vi "Thread_Conductor.vi"(5 "Ce VI":refnum<vi>, 7 "Display":refnum<vi>, 8 "entrée d'erreur (pas d'erreur)":errorcluster, 11 "File d'attente en entrée":refnum<queue>) -> (0 "error out":errorcluster caption="sortie d'erreur", 2 "Data Cluster":T1, 3 "File d'attente en sortie":refnum<queue>)   [LabVIEW 2020]
doc: "Conductor thread qui va gérer les opération"
uses:
  support/Message Queue/Message Cluster.ctl
  controls/UI Data.ctl
  support/Message Queue/All Message Queues.ctl
  Calculatrice/controls/ctrl_UI_Ref.ctl
  Calculatrice/controls/ctrl_Ref.ctl
  Calculatrice/controls/ctrl_Event_Ref.ctl
  controls/Ctrl_RefPad.ctl
  support/Message Queue/Enqueue Message (Single).vi
  <vilib>/Utility/error.llb/Error Cluster From Error Code.vi
  <vilib>/ErrorRing/Error Ring.xnode
  support/Message Queue/Message Queue.lvlib
  support/User Event - Stop/User Event - Stop.lvlib
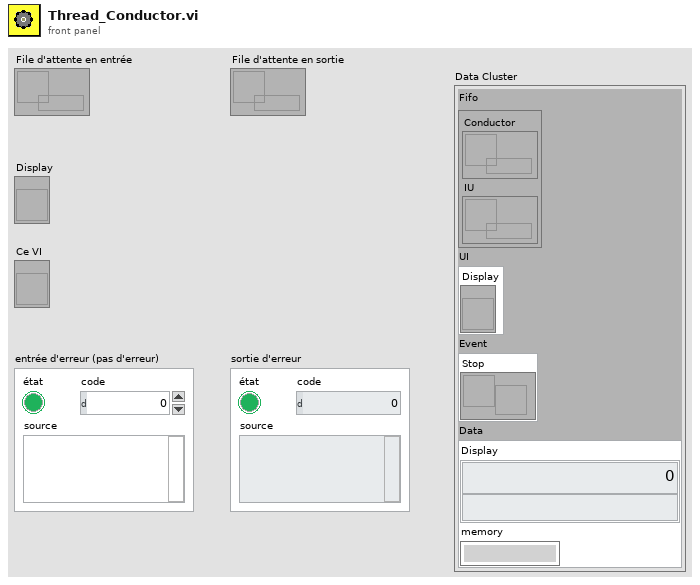
[diagram p1: front panel]
types:
  T1 = typedef "UI Data.ctl" = cluster{"Fifo":T2, "UI":T3, "Event":cluster{"Stop":refnum<user-event>}, "Data":cluster{"Display":cluster{"Num":dbl, "Char":string}, "memory":string}}
  T2 = typedef "Message Queue.lvlib/All Message Queues.ctl" = cluster{"Conductor":refnum<queue>, "IU":refnum<queue>}
  T3 = typedef "ctrl_UI_Ref.ctl" = cluster{"Display":refnum<vi>}
  T4 = typedef "ctrl_Ref.ctl" = cluster{"Fifo":T2, "Event":T5, "UI":T3}
  T5 = typedef "ctrl_Event_Ref.ctl" = cluster{"Stop Event":refnum<user-event>}
  T6 = typedef "Ctrl_RefPad.ctl" = cluster{"BTN_Ref":refnum<vi>, "CharPad":string}
  T7 = cluster{"état":bool, "code":i32, "source":string}
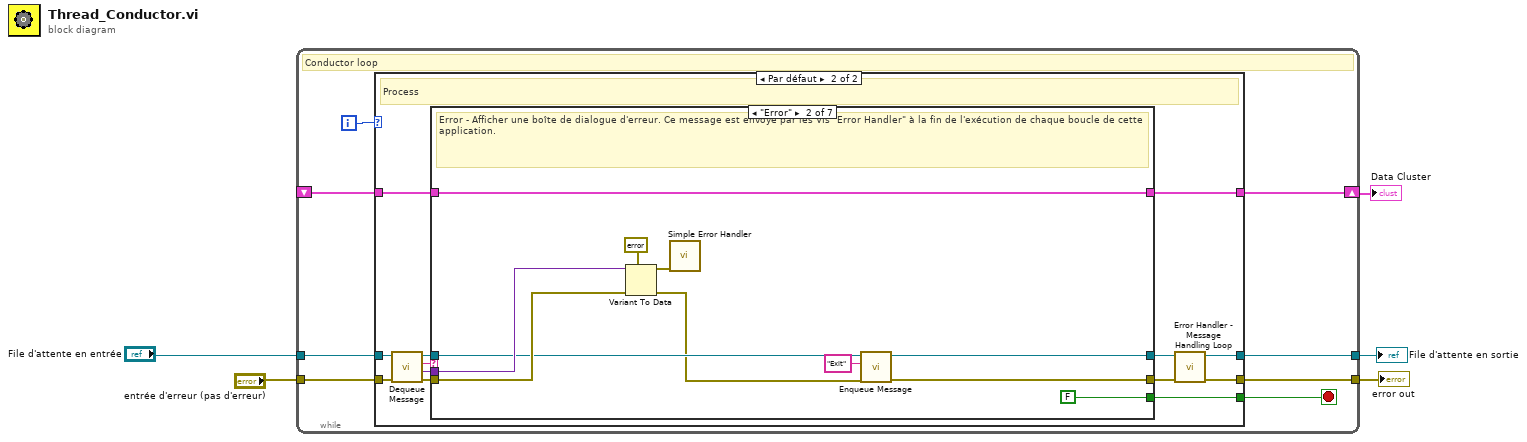
[diagram p0: block diagram]
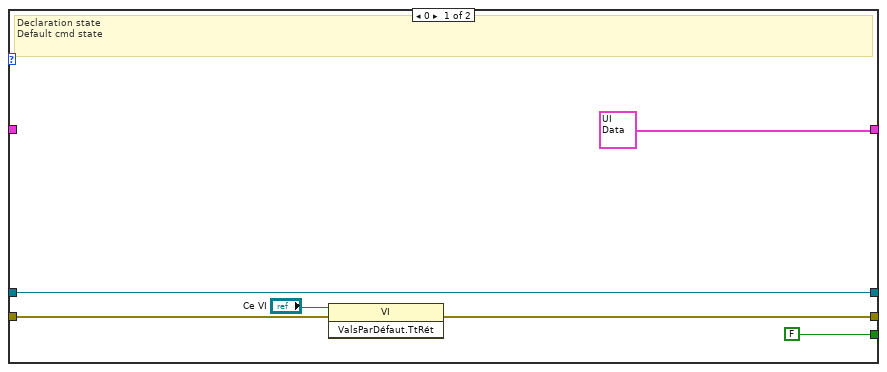
[diagram p2: hidden frame]
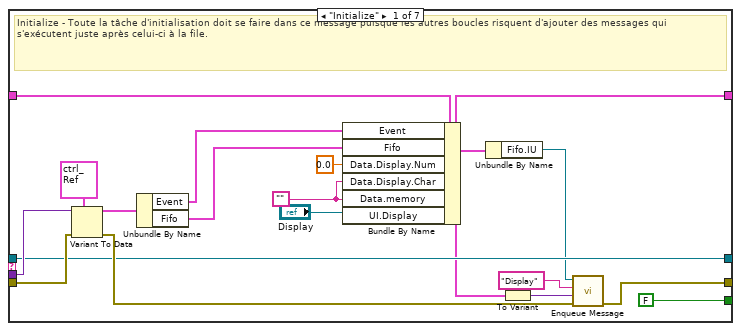
[diagram p3: hidden frame]
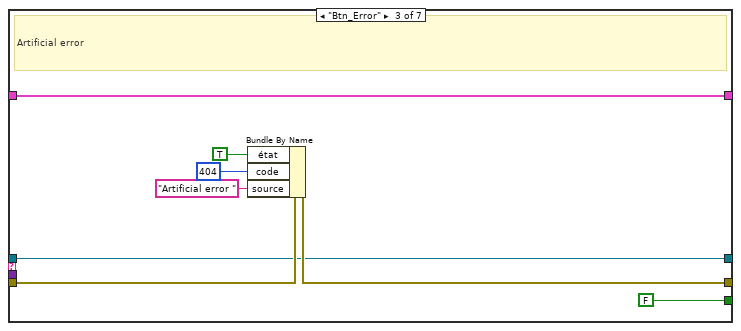
[diagram p4: hidden frame]
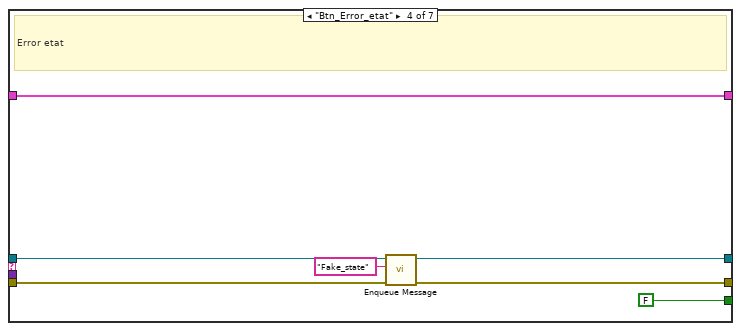
[diagram p5: hidden frame]
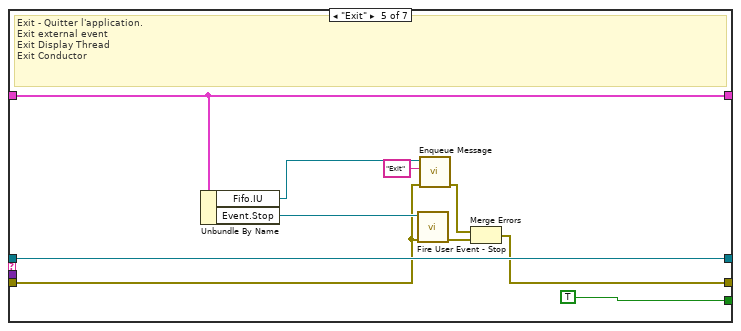
[diagram p6: hidden frame]
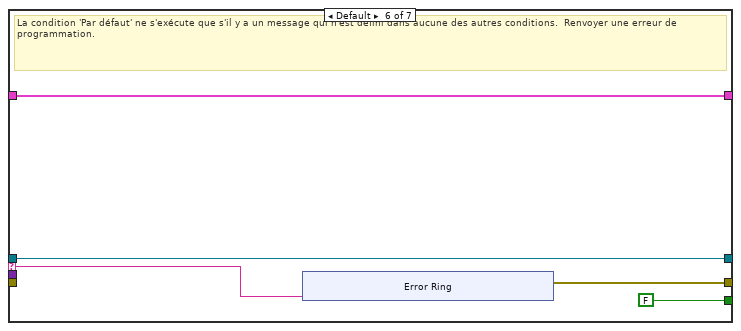
[diagram p7: hidden frame]
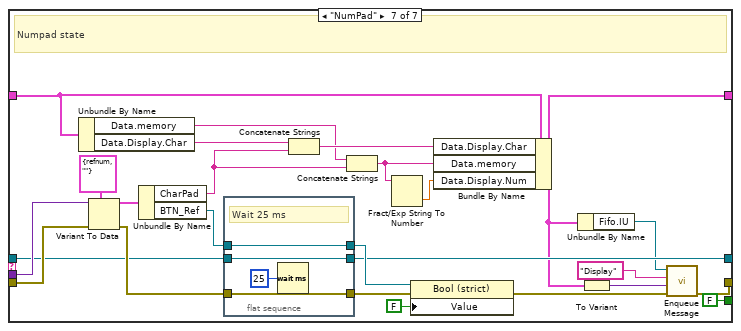
[diagram p8: hidden frame]
diagram:
  n1 = while {
    tunnel: "File d'attente en entrée" -> [w9]
    shift-right: [w12] -> w3
    shift-left: _ -> [w13]
    tunnel: "entrée d'erreur (pas d'erreur)" -> [w10]
    tunnel: [w8] -> w1
    tunnel: [w7] -> w4
    i -> [w6]
    stop <- w11 stop-if-true
    # "Conductor loop"
    n2 = case shown="Par défaut" w6 {
      tunnel: w13 -> [_ w32]
      tunnel: [T1 {"Fifo"={"Conductor"=refnum, "IU"=refnum}, "UI"={"Display"=refnum}, "Event"={"Stop"=refnum}, "Data"={"Display"={"Num"=0.0, "Char"=""}, "memory"=""}} ("Data Cluster") w31] -> w12
      tunnel: [FALSE w30] -> w11
      tunnel: w10 -> [w15 w29]
      tunnel: w9 -> [w18 w25]
      tunnel: [w14 w23] -> w8
      tunnel: [w18 w20] -> w7
      frame 0 {
        # "Declaration state\nDefault cmd state"
        n3 = invoke class="VI" method="ValsParDéfaut.TtRét"(reference="Ce VI", error in=w15) -> (error out=w14:errorcluster)  [unwired: 1 in, 2 out]
      }
      frame Default {
        # "Process"
        n4 = call "Dequeue Message.vi"("error in (no error)"=w29, "File d'attente de messages"=w25) -> ("error out"=w28:T7, "Données de message"=w26:variant, "Message"=w27:string, "File d'attente de message dup."=w24:refnum<queue>)  [unwired: 6 in]
        n5 = case "Conditions des messages" shown="\"Error\"" w27 {
          selector: w27 -> [_ _ _ _ _ w89 _]
          tunnel: w24 -> [w36 w55 w63 w72 w83 w87 w107]
          tunnel: w28 -> [w47 w61 w69 w75 w80 _ w123]
          tunnel: [w50 w52 w67 w74 w79 w90 w119] -> w22
          tunnel: w32 -> [w49 w60 w68 w76 w85 w91 w118]
          tunnel: [w34 w60 w68 w76 w85 w91 w100] -> w31
          tunnel: [FALSE FALSE FALSE FALSE TRUE FALSE FALSE] -> w30
          tunnel: w26 -> [w46 w59 _ _ _ _ w122]
          tunnel: [w36 w54 w63 w73 w83 w87 w101] -> w21
          frame "Initialize" {
            w43 = ""
            # "Initialize - Toute la tâche d'initialisation doit se faire dans ce message puisque les autres boucles risquent d'ajouter des messages qui s'exécutent juste après celui-ci à la file."
            n6 = Variant To Data(error in=w47, type=T4 {"Fifo"={"Conductor"=refnum, "IU"=refnum}, "Event"={"Stop Event"=refnum}, "UI"={"Display"=refnum}} ("Ref"), Variant=w46) -> (data=w40:T4, error out=w45:errorcluster)
            n7 = Unbundle By Name(w40) -> ("Event"=w38:T5, "Fifo"=w39:T2)
            n8 = Bundle By Name(cluster=w49, "Event"=w38, "Fifo"=w39, "Data.Display.Num"=0.0, "Data.Display.Char"=w43, "Data.memory"=w43, "UI.Display"="Display") -> (w34:T1)
            n9 = Unbundle By Name(w34) -> ("Fifo.IU"=w33:refnum<queue>)
            n10 = To Variant(anything=w34) -> (Variant=w35:variant)
            n11 = call-poly "Enqueue Message.vi"("error in (no error)"=w45, "Données de message"=w35, "Message"="Display", "File d'attente de messages"=w33) -> ("error out"=w50:T7)  [unwired: 6 in, 1 out]
          }
          frame "Error" {
            # "Error - Afficher une boîte de dialogue d'erreur. Ce message est envoyé par les VIs \"Error Handler\" à la fin de l'exécution de chaque boucle de cette application."
            n12 = Variant To Data(error in=w61, type=errorcluster {"status"=FALSE, "code"=0, "source"=""} ("error constant"), Variant=w59) -> (data=w57:errorcluster, error out=w53:errorcluster)
            n13 = call <vilib>:"Simple Error Handler.vi"("error in (no error)"=w57) -> ()  [unwired: 4 in, 5 out]
            n14 = call-poly "Enqueue Message.vi"("error in (no error)"=w53, "Message"="Exit", "File d'attente de messages"=w55) -> ("error out"=w52:T7, "File d'attente de message dup."=w54:refnum<queue>)  [unwired: 7 in]
          }
          frame "Btn_Error" {
            # "Artificial error"
            n15 = Bundle By Name(cluster=w69, "état"=TRUE, "code"=404, "source"="Artificial error ") -> (w67:T7)
          }
          frame "Btn_Error_etat" {
            # "Error etat"
            n16 = call-poly "Enqueue Message.vi"("error in (no error)"=w75, "Message"="Fake_state", "File d'attente de messages"=w72) -> ("error out"=w74:T7, "File d'attente de message dup."=w73:refnum<queue>)  [unwired: 7 in]
          }
          frame "Exit" {
            # "Exit - Quitter l'application.\nExit external event\nExit Display Thread\nExit Conductor"
            n17 = Unbundle By Name(w85) -> ("Fifo.IU"=w81:refnum<queue>, "Event.Stop"=w84:refnum<user-event>)
            n18 = call "Fire User Event - Stop.vi"("error in (no error)"=w80, "Événement utilisateur - Arrêt"=w84) -> ("error out"=w82:T7)  [unwired: 9 in]
            n19 = call-poly "Enqueue Message.vi"("error in (no error)"=w80, "Message"="Exit", "File d'attente de messages"=w81) -> ("error out"=w78:T7)  [unwired: 7 in, 1 out]
            n20 = Merge Errors(w78, w82) -> (w79:errorcluster)
          }
          frame Default {
            # "La condition 'Par défaut' ne s'exécute que s'il y a un message qui n'est défini dans aucune des autres conditions.  Renvoyer une erreur de programmation."
            n21 = xnode ("Error Ring")("paramètre 0"=w89) -> ("sortie d'erreur"=w90:errorcluster)
          }
          frame "NumPad" {
            # "Numpad state"
            n22 = Unbundle By Name(w118) -> ("Data.memory"=w115:string, "Data.Display.Char"=w117:string)
            n23 = Variant To Data(error in=w123, type=T6 {"BTN_Ref"=refnum, "CharPad"=""} ("cluster"), Variant=w122) -> (data=w111:T6, error out=w108:errorcluster)
            n24 = Unbundle By Name(w111) -> ("CharPad"=w110:string, "BTN_Ref"=w109:refnum<vi>)
            n25 = flat-sequence {
              tunnel: w109 -> [w126]
              tunnel: [w126] -> w105
              tunnel: w108 -> [w125]
              tunnel: w107 -> [w124]
              tunnel: [w125] -> w106
              tunnel: [w124] -> w101
              frame #0 {
                # "Wait 25 ms"
                n26 = Wait (ms)(milliseconds to wait=u32 25 ("attente (ms)")) -> ()  [unwired: 1 out]
              }
            }
            n27 = Concatenate Strings(w117, w110) -> (w116:string)
            n28 = Concatenate Strings(w115, w110) -> (w114:string)
            n29 = Fract/Exp String To Number(string=w114) -> (number=w113:dbl)  [unwired: 3 in, 1 out]
            n30 = property class="Bool (strict)"(reference=w105, error in=w106, "Value"=FALSE ("Valeur")) -> (error out=w104:errorcluster)  [unwired: 1 out]
            n31 = Bundle By Name(cluster=w118, "Data.Display.Char"=w116, "Data.memory"=w114, "Data.Display.Num"=w113) -> (w100:T1)
            n32 = Unbundle By Name(w100) -> ("Fifo.IU"=w99:refnum<queue>)
            n33 = To Variant(anything=w100) -> (Variant=w102:variant)
            n34 = call-poly "Enqueue Message.vi"("error in (no error)"=w104, "Données de message"=w102, "Message"="Display", "File d'attente de messages"=w99) -> ("error out"=w119:T7)  [unwired: 6 in, 1 out]
          }
        }
        n35 = call "Error Handler - Message Handling Loop.vi"("error in (no error)"=w22, "File d'attente de messages"=w21) -> ("erreur en entrée dup."=w23:T7, "File d'attente de message dup."=w20:refnum<queue>)  [unwired: 8 in]
      }
    }
  }
  "File d'attente en sortie" <- w4
  "Data Cluster" <- w3
  "error out" <- w1
